vi "PXDAC4800_SessionStreamGetProgressXD48.vi"(0 "StreamSessionHandle":u32, 5 "Flags":i32) -> (4 "Status":i32, 6 "StreamProgressInfo":T1)   [LabVIEW 2016]
uses:
  PXDAC4800.dll
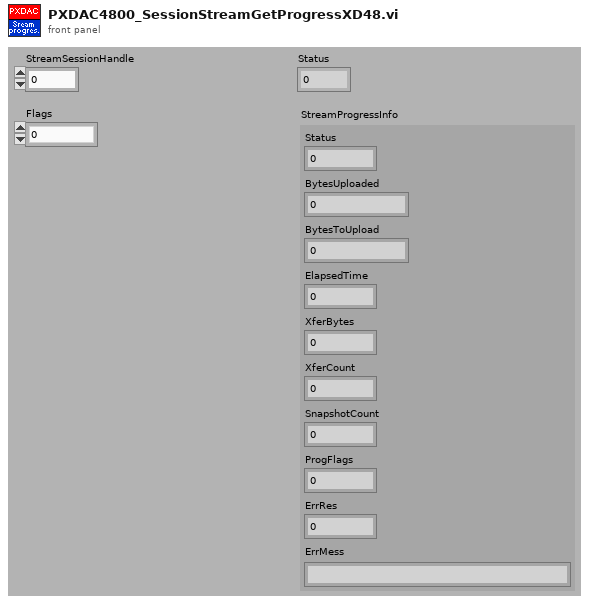
[diagram p1: front panel]
types:
  T1 = cluster{"Status":i32, "BytesUploaded":dbl, "BytesToUpload":dbl, "ElapsedTime":u32, "XferBytes":u32, "XferCount":u32, "SnapshotCount":u32, "ProgFlags":i32, "ErrRes":i32, "ErrMess":string}
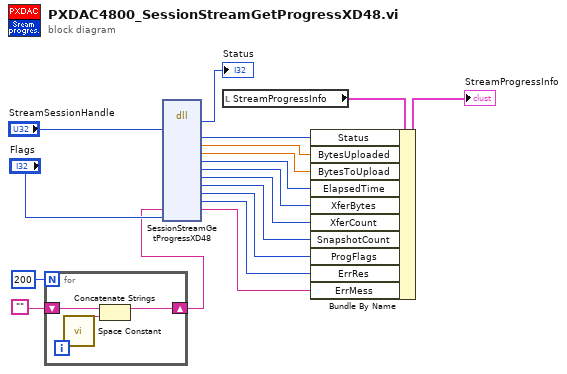
[diagram p0: block diagram]
diagram:
  n1 = for {
    N: 200 -> [_]
    shift-right: [w19] -> w2
    shift-left: "" -> [w20]
    n2 = call <vilib>:"Space Constant.vi"() -> ("String"=w21:string)
    n3 = Concatenate Strings(w20, w21) -> (w19:string)
  }
  n4 = dll-call lib="PXDAC4800.dll" fn="SessionStreamGetProgressXD48"("StreamSessHandle"="StreamSessionHandle", "ErrMess"=w2, "Flags"="Flags") -> (→"Status":i32, "Status"=w15:i32, "BytesUploaded"=w14:dbl, "BytesToUpload"=w13:dbl, "ElapsedTimeMs"=w12:u32, "XferBytes"=w11:u32, "XferCount"=w10:u32, "SsCount"=w9:u32, "ProgFlags"=w8:i32, "ErrRes"=w7:i32, "ErrMess"=w4:string)  [unwired: 14 in, 2 out]
  n5 = local read "StreamProgressInfo"() -> (w16:T1)
  n6 = Bundle By Name(cluster=w16, "Status"=w15, "BytesUploaded"=w14, "BytesToUpload"=w13, "ElapsedTime"=w12, "XferBytes"=w11, "XferCount"=w10, "SnapshotCount"=w9, "ProgFlags"=w8, "ErrRes"=w7, "ErrMess"=w4) -> (→"StreamProgressInfo":T1)
